vi "連續移動生成.vi"() -> ()   [LabVIEW 2015]
panel:
  out "XY Graph 2":cluster{"Y":dbl[], "Y":dbl[]}[](graph)
  out "XY Graph":cluster{dbl[], dbl[]}(graph)
  in  "Array":T1(array[cluster])
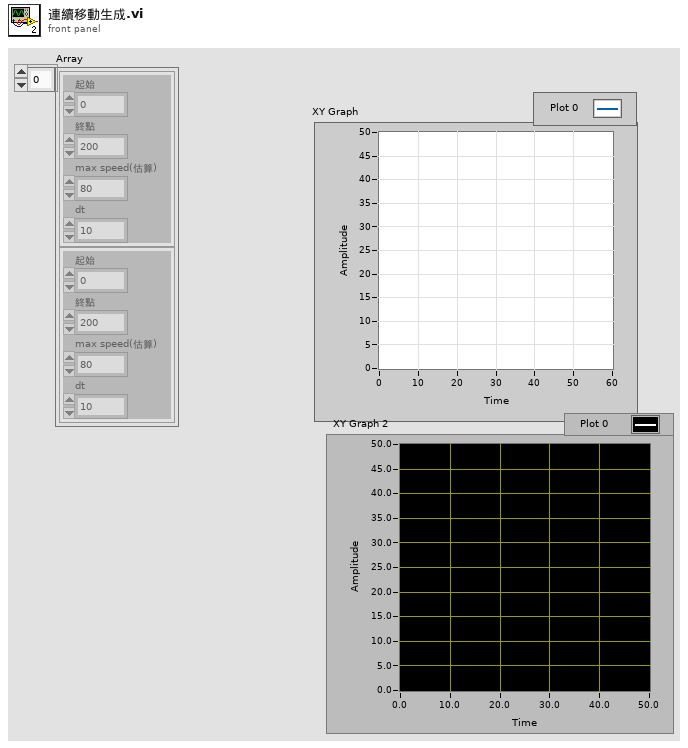
[diagram p1: front panel]
types:
  T1 = cluster{"起始":dbl, "終點":dbl, "max speed(估算)":dbl, "dt":dbl}[]
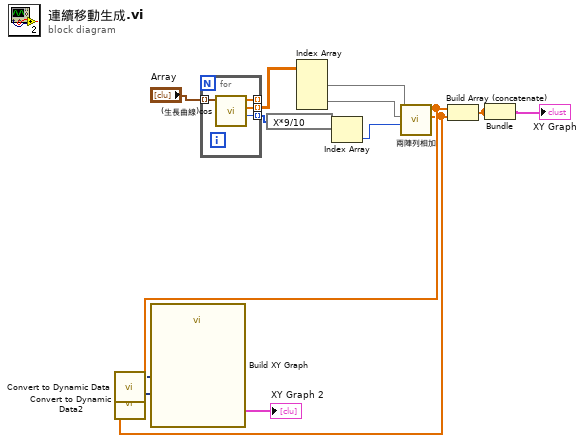
[diagram p0: block diagram]
diagram:
  n1 = for {
    tunnel: "Array" -> [w18] mode=indexing
    tunnel: [w17] -> w12 mode=indexing
    tunnel: [w16] -> w13 mode=indexing
    tunnel: [w15] -> _ mode=indexing
    n2 = call "(生長曲線)cos.vi"("目標in"=w18) -> ("次數"=w16:i32, "距離曲線(cm)"=w17:dbl[], "speed曲線(cm/s)"=w15:dbl[])  [unwired: 8 in]
  }
  n3 = expression code="X*9/10"(w13) -> (w11:i32[])
  n4 = Index Array(array=w12) -> (element #1=w8:dbl[], element #2=w9:dbl[])  [unwired: 4 in]
  n5 = Index Array(array=w11) -> (element=w10:i32)  [unwired: 1 in]
  n6 = call "兩陣列相加.vi"("INDEX"=w10, "++Y"=w9, "++X"=w8) -> ("Y array"=w2:dbl[], "X array"=w4:dbl[])  [unwired: 7 in]
  n7 = call "Convert to Dynamic Data"("Array"=w4) -> ("Dynamic Data Type"=w3:dynamicdata)  [unwired: 3 in]
  n8 = call "Convert to Dynamic Data2"("Array"=w2) -> ("Dynamic Data Type"=w1:dynamicdata)  [unwired: 3 in]
  n9 = call "Build XY Graph"("Y Input"=w1, "X Input"=w3) -> ("XY Graph"=→"XY Graph 2":cluster{"X":dbl[], "Y":dbl[]}[])  [unwired: 8 in, 1 out]
  n10 = Build Array (concatenate)(w4, w2) -> (w7:dbl[])
  n11 = Bundle(w7, w7) -> (→"XY Graph":cluster{dbl[], dbl[]})  [unwired: 1 in]
